vi "squareOrIntersection2.vi"(6 "Parâmetros Ini":T3={"Gyro Port"=0, "Sensor - Left"=3, "Sensor - Right"=2, "     Color \nSensor Port"=1, "Kp Front"=0.5, "Motor speed"=-15, "Distance to street"=0.0, "Motor speed turns"=16, "Kp Curvas"=0.0} {"Kp Front" format="%.3f"; "Color \nSensor Port" items=["Port 1", "Port 2", "Port 3", "Port 4"]; "Sensor - Right" items=["Port 1", "Port 2", "Port 3", "Port 4"]; "Sensor - Left" items=["Port 1", "Port 2", "Port 3", "Port 4"]; "Gyro Port" items=["Port 1", "Port 2", "Port 3", "Port 4"]}, 10 "NXT/EV3":T2) -> (0 "Detected Color":T1, 1 "CS":enum16{"Street", "Intersection", "End", "Stop"}(ring), 3 "NXT/EV3 2":T2)   [LabVIEW 2016]
uses:
  <vilib>/NXT/Subs/LVHSConnector.ctl
  <vilib>/NXT/LegoClasses/BrickReference/BrickReference.lvclass
  <vilib>/NXT/Subs/ColorSensorColors.ctl
  parametros.ctl
  <vilib>/NXT/Block Support/NXT_InputPort.ctl
  <vilib>/NXT/Block Support/NXT_OutputPort.ctl
  <vilib>/NXT/NXTIO Xnodes/NXTIONodeSubVIs/NXTStopMotors.vi
  <vilib>/NXT/NXTIO Xnodes/AddressXNode/NXTIOAddress.xnode
  <vilib>/NXT/NXTIO Xnodes/NXTIOXNode/NXTIO.xnode
panel:
  in  "Contador de cores 1":dbl
  out "Numeric":i32
  out "Array":T1[](array[typedef])
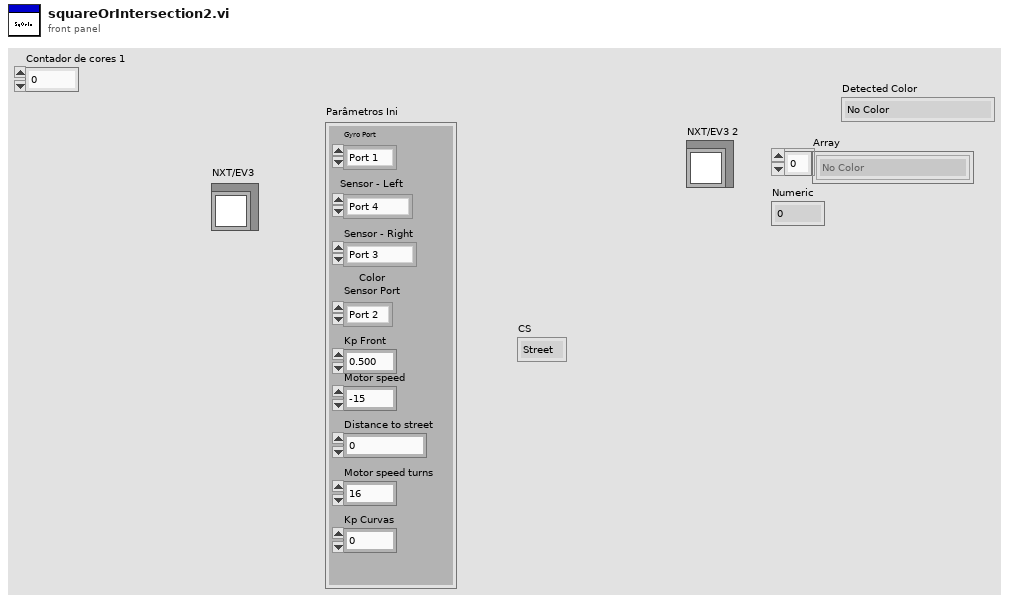
[diagram p1: front panel]
types:
  T1 = typedef "ColorSensorColors.ctl" = enum16{"No Color", "Black", "Blue", "Green", "Yellow", "Red", "White", "Brown"}
  T2 = typedef "LVHSConnector.ctl" = refnum<class "BrickReference.lvclass">
  T3 = typedef "parametros.ctl" = cluster{"Gyro Port":T4, "Sensor - Left":T4, "Sensor - Right":T4, "     Color \nSensor Port":T4, "Kp Front":dbl, "Motor speed":i32, "Distance to street":dbl, "Motor speed turns":i32, "Kp Curvas":dbl}
  T4 = typedef "NXT_InputPort.ctl" = u32
  T5 = enum16{"Street", "Intersection", "End", "Stop", "Square", "Delivery", "Empty"}
  T6 = typedef "NXT_OutputPort.ctl" = u8
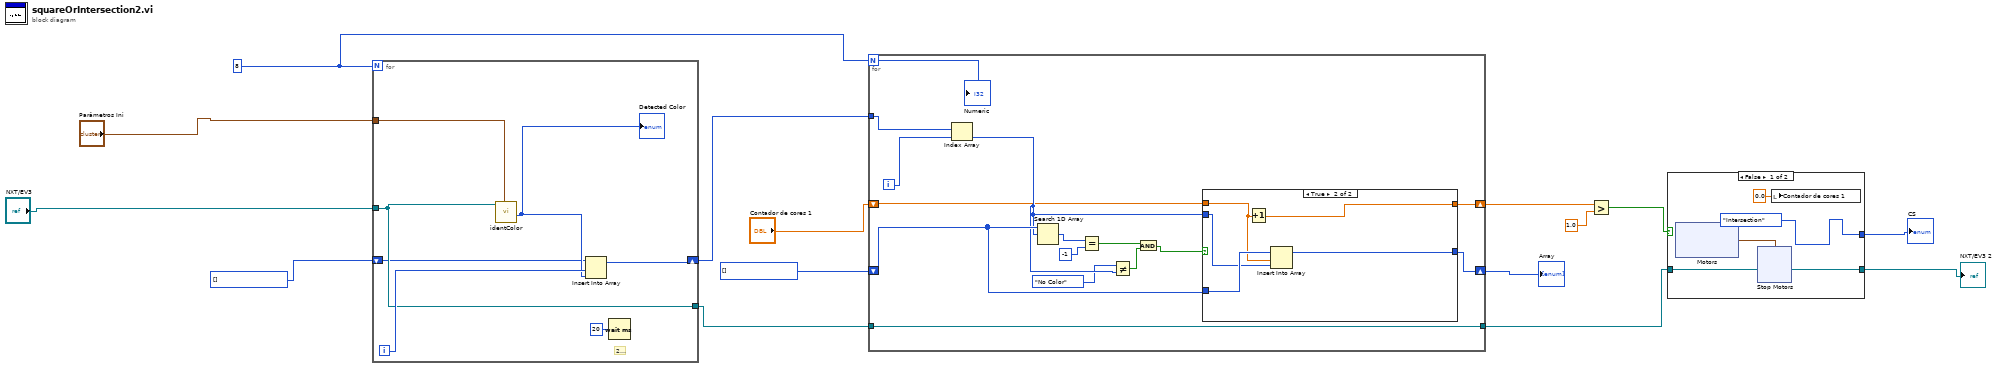
[diagram p0: block diagram]
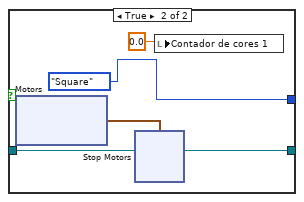
[diagram p2: hidden frame]
diagram:
  w3 = T1[] [] items=["No Color", "Black", "Blue", "Green", "Yellow", "Red", "White", "Brown"] ("array")
  w5 = T1[] [] items=["No Color", "Black", "Blue", "Green", "Yellow", "Red", "White", "Brown"] ("array")
  w14 = 8
  n1 = for {
    N: w14 -> [_]
    shift-right: [w21] -> w15
    shift-left: w5 -> [w16]
    tunnel: "Parâmetros Ini" -> [w19]
    tunnel: [w17] -> w9
    tunnel: "NXT/EV3" -> [w17]
    i -> [w22]
    # "250"
    n2 = call "identColor.vi"("Parâmetros Ini"=w19, "NXT/EV3"=w17) -> ("Collor"=w20:T1)  [unwired: 8 in, 1 out]
    "Detected Color" <- w20
    n3 = Insert Into Array(array=w16, index=w22, new element=w20) -> (w21:T1[])
    n4 = Wait (ms)(milliseconds to wait=u32 20) -> ()  [unwired: 1 out]
  }
  n5 = for {
    N: w14 -> [w31]
    tunnel: w15 -> [w36]
    shift-right: [w33] -> w4
    shift-left: w3 -> [w34]
    tunnel: [w32] -> w7
    tunnel: w9 -> [w32]
    shift-right: [w30] -> w2
    shift-left: "Contador de cores 1" -> [w23]
    i -> [w37]
    n6 = Index Array(array=w36, index=w37) -> (element=w26:T1)
    n7 = Search 1D Array(1D array=w34, element=w26) -> (index of element=w27:i32)  [unwired: 1 in]
    n8 = Equal?(x=w27, y=-1) -> (x = y?=w29:bool)
    n9 = Not Equal?(x=ColorSensorColors."No Color", y=w26) -> (x != y?=w28:bool)
    n10 = And(x=w29, y=w28) -> (x .and. y?=w24:bool)
    n11 = case shown="True" w24 {
      tunnel: w34 -> [w39 w44]
      tunnel: w26 -> [_ w43]
      tunnel: [w39 w42] -> w33
      tunnel: [w38 w40] -> w30
      tunnel: w23 -> [w38 w41]
      frame False {
      }
      frame True {
        n12 = Increment(x=w41) -> (x+1=w40:dbl)
        n13 = Insert Into Array(array=w44, index=w41, new element=w43) -> (w42:T1[])
      }
    }
    "Numeric" <- w31
  }
  "Array" <- w4
  n14 = Greater?(x=w2, y=1.0) -> (0:w11:bool)
  n15 = case shown="False" w11 {
    tunnel: [T5."Intersection" ("CS") T5."Square" ("CS")] -> w10
    tunnel: [w48 w58] -> w8
    tunnel: w7 -> [w48 w58]
    frame False {
      n16 = xnode "Motors"() -> ("Motor"=w47:cluster{"Port":T6, "Port":T6})
      n17 = xnode "Stop Motors"("Motors"=w47) -> ()  [unwired: 1 in, 1 out]
      n18 = local write "Contador de cores 1"(0.0 ("Contador de cores 1")) -> ()
    }
    frame True {
      n19 = xnode "Motors"() -> ("Motor"=w57:cluster{"Port":T6, "Port":T6})
      n20 = xnode "Stop Motors"("Motors"=w57) -> ()  [unwired: 1 in, 1 out]
      n21 = local write "Contador de cores 1"(0.0 ("Contador de cores 1")) -> ()
    }
  }
  "NXT/EV3 2" <- w8
  "CS" <- w10
